vi "Brower View Rename.vi"(8 "error in (no error)":errorcluster, 10 "PreviousName":string, 11 "Brower View in":refnum<class "Brower View.lvclass">) -> (0 "error out":errorcluster, 2 "New Name Out":string, 3 "Brower View out":refnum<class "Brower View.lvclass">)   [LabVIEW 2015, in "Brower View.lvclass"]
uses:
  Brower View.lvclass
  Type Definition/Brower State Variable.ctl
panel:
  in  "Cancel":bool
  in  "Restore":bool
  in  "Sure":bool
  in  "New Name":string
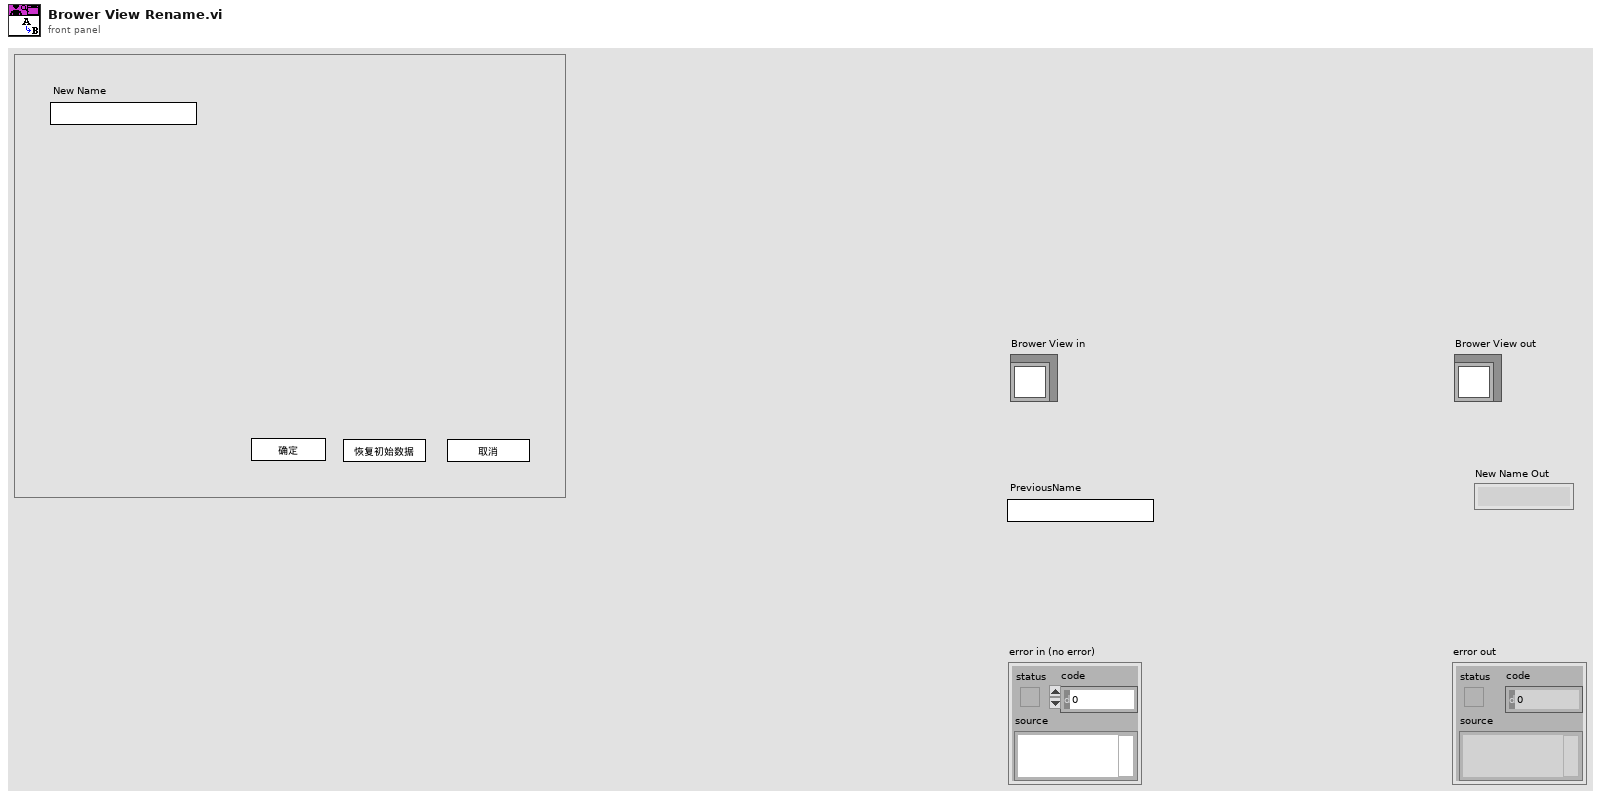
[diagram p1: front panel]
types:
  T1 = typedef "Brower View.lvclass/Brower State Variable.ctl" = enum16{"PanelOn", "Rename", "PanelOff"}
  T2 = enum32{"Invalid", "Standard", "Closed", "Hidden", "Minimized", "Maximized"}
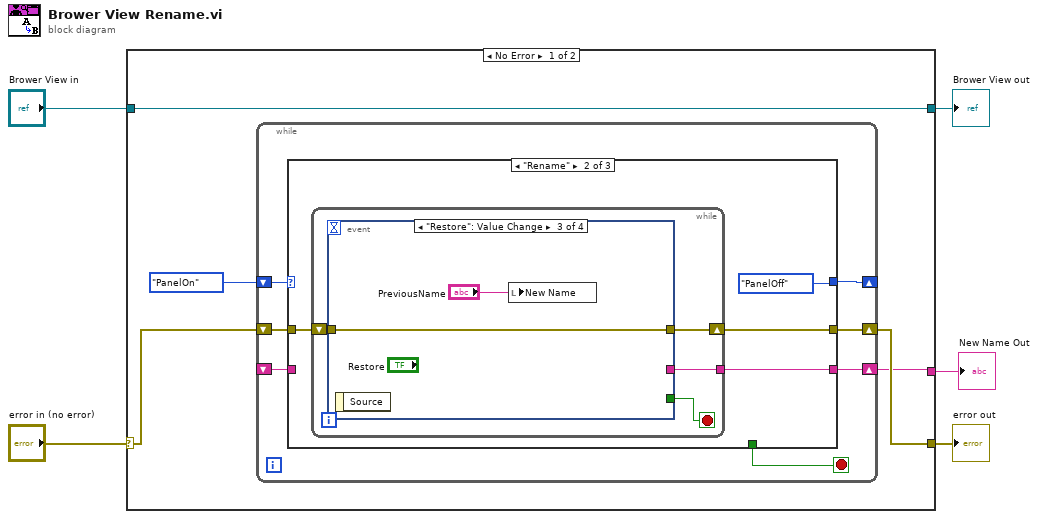
[diagram p0: block diagram]
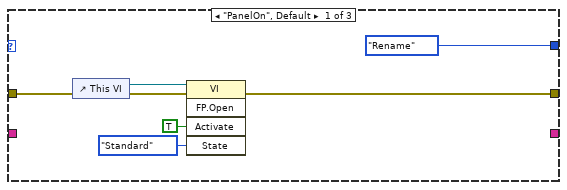
[diagram p2: hidden frame]
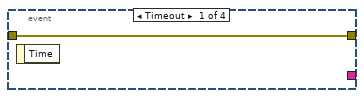
[diagram p3: hidden frame]
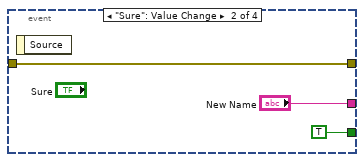
[diagram p4: hidden frame]
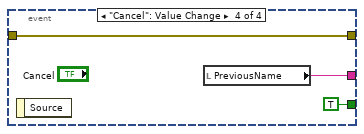
[diagram p5: hidden frame]
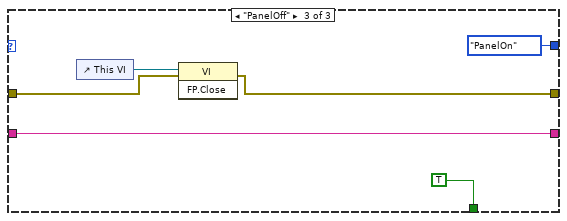
[diagram p6: hidden frame]
diagram:
  n1 = case shown="No Error" "error in (no error)" {
    selector: "error in (no error)" -> [w8 w48]
    tunnel: [w7 w48] -> w4
    tunnel: [w10 w47] -> w2
    tunnel: "Brower View in" -> [w10 w47]
    tunnel: [w6 _] -> w1
    frame No Error {
      n2 = while {
        shift-right: [w15] -> w7
        shift-left: w8 -> [w16]
        shift-right: [w13] -> _
        shift-left: Brower_State_Variable."PanelOn" -> [w17]
        shift-right: [w14] -> w6
        shift-left: _ -> [w11]
        stop <- w12 stop-if-true
        n3 = case shown="\"Rename\"" w17 {
          tunnel: w16 -> [w22 w27 w42]
          tunnel: [w19 w26 w41] -> w15
          tunnel: [_ w25 w44] -> w14
          tunnel: [Brower_State_Variable."Rename" Brower_State_Variable."PanelOff" Brower_State_Variable."PanelOn"] -> w13
          tunnel: [_ _ TRUE] -> w12
          tunnel: w11 -> [_ _ w44]
          frame "PanelOn", Default {
            n4 = control-ref of="This VI"() -> (w23:refnum<vi>)
            n5 = invoke class="VI" method="FP.Open"(reference=w23, error in=w22, "Activate"=TRUE ("Activate?"), "State"=T2."Standard") -> (error out=w19:errorcluster)  [unwired: 1 in, 4 out]
          }
          frame "Rename" {
            n6 = while {
              tunnel: [w29] -> w25
              shift-right: [w30] -> w26
              shift-left: w27 -> [w31]
              stop <- w28 stop-if-true
              n7 = event shown="[2] \"Restore\": Value Change" {
                selector: _ -> [_ _ _ _]
                dyn-events: _ -> [_ _ _ _]
                timeout: _ -> [_ _ _ _]
                tunnel: w31 -> [w32 w35 w37 w40]
                tunnel: [w32 w35 w37 w40] -> w30
                tunnel: [_ "New Name" _ w39] -> w29
                tunnel: [_ TRUE _ TRUE] -> w28
                event Timeout {
                  n8 = event-data() -> ()  [unwired: 1 in, 1 out]
                }
                event "Sure": Value Change {
                  n9 = event-data() -> ()  [unwired: 1 in, 1 out]
                }
                event "Restore": Value Change {
                  n10 = event-data() -> ()  [unwired: 1 in, 1 out]
                  n11 = local write "New Name"("PreviousName") -> ()
                }
                event "Cancel": Value Change {
                  n12 = event-data() -> ()  [unwired: 1 in, 1 out]
                  n13 = local read "PreviousName"() -> (w39:string)
                }
              }
            }
          }
          frame "PanelOff" {
            n14 = control-ref of="This VI"() -> (w43:refnum<vi>)
            n15 = invoke class="VI" method="FP.Close"(reference=w43, error in=w42) -> (error out=w41:errorcluster)  [unwired: 1 in, 2 out]
          }
        }
      }
    }
    frame Error {
    }
  }
  "error out" <- w4
  "Brower View out" <- w2
  "New Name Out" <- w1
